vi "Create Arbitrary Waveform_Corr6.vi"(8 "error in (no error)":errorcluster, 10 "Waveform Name (\"wave1\")":string="wave1", 11 "VISA resource name":refnum<visa-resource-name>="USB0::0xF4EC::0x1101::SDG6XEBC5R0119::INSTR") -> ()   [LabVIEW 2018]
doc: "Creates and saves an arbitrary (user-defined) waveform in non-volatile memory, then selects it for output."
uses:
  <vilib>/Utility/file.llb/Read From Spreadsheet File (I64).vi
panel:
  out "error out":errorcluster
  out "VISA resource name out":refnum<visa-resource-name>
  out "Attempts":i32
  in  "WFM Source":u16(ring) items=["Single file", "Split files", "Array"]
  in  "WFM Path":path=path "C:/Data/_SoftDevelopment/SDG6000/PMHtst.txt"
  in  "WFM (Column) Number":i32
  in  "WFM Length":i32=15
  in  "Arbitrary Numeric Waveform Data":dbl[](array[numeric])=[1000.0, 2000.0, 3000.0, 4000.0, 5000.0, 6000.0, 7000.0, 8000.0]
  # "Same vi as with suppliers example,\nbut incorrect negativ case removed.\nInstead calculating twos complement\nexplicitly for negative values.\nThe input range for ARB data is\n-32768..+32767"
  # "C1 hardcoded as needs to have a channel assigned to be uploaded. \nCan then be used for either channel"
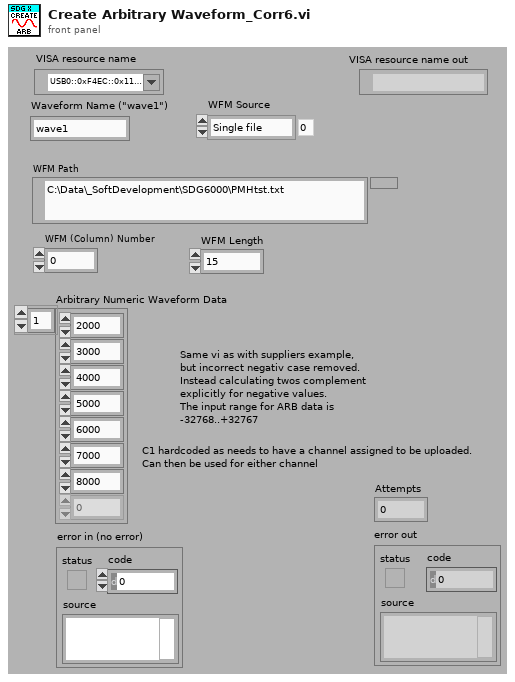
[diagram p1: front panel]
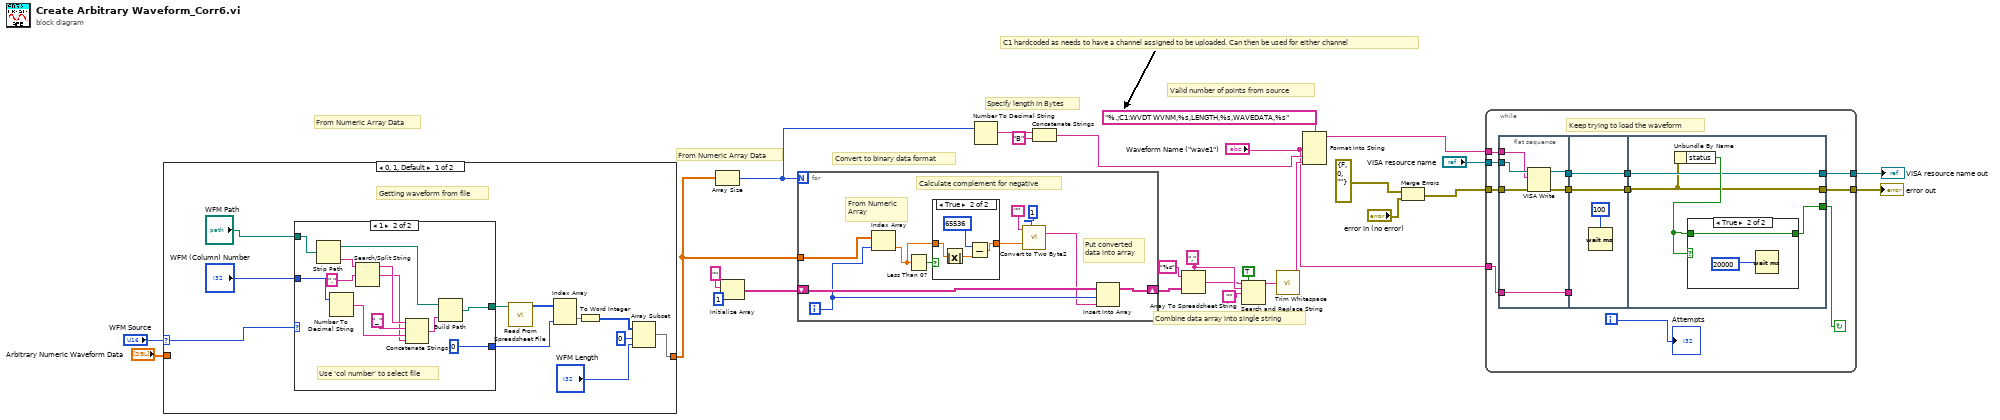
[diagram p0: block diagram]
diagram:
  w19 = ","
  # "C1 hardcoded as needs to have a channel assigned to be uploaded. Can then be used for either channel"
  # "From Numeric Array Data"
  # "From Numeric Array Data"
  # "Specify length in Bytes"
  # "Combine data array into single string"
  # "Valid number of points from source"
  # "Convert to binary data format"
  n1 = case shown="0, 1, Default" "WFM Source" {
    selector: "WFM Source" -> [w33 _]
    tunnel: [w28 w53] -> w8
    tunnel: "Arbitrary Numeric Waveform Data" -> [_ w53]
    frame 0, 1, Default {
      # "Getting waveform from file"
      n2 = case shown="1" w33 {
        tunnel: "WFM Path" -> [w40 w52]
        tunnel: "WFM (Column) Number" -> [w39 w49]
        tunnel: [w40 w42] -> w31
        tunnel: [w39 0 ("x")] -> w30
        frame 0, Default {
          # "File contains multiple wfms"
        }
        frame 1 {
          # "Use 'col number' to select file"
          n3 = Strip Path(path=w52) -> (stripped path=w44:path, name=w50:string)
          n4 = Number To Decimal String(number=w49) -> (decimal integer string=w46:string)  [unwired: 1 in]
          n5 = Search/Split String(string=w50, search string/char (-)=".") -> (substring before match=w48:string, match + rest of string=w45:string)  [unwired: 1 in, 1 out]
          n6 = Concatenate Strings(w48, "_", w46, w45) -> (w43:string)
          n7 = Build Path(base path=w44, name or relative path=w43) -> (appended path=w42:path)
        }
      }
      n8 = call-poly <vilib>:"Read From Spreadsheet File.vi"("file path (dialog if empty)"=w31) -> ("all rows"=w32:i64[][])  [unwired: 6 in, 4 out]
      n9 = Index Array(array=w32, index (col)=w30) -> (element=w29:i64[])  [unwired: 1 in]
      n10 = To Word Integer(number=w29) -> (16bit integer=w38:i16[])
      n11 = Array Subset(array=w38, index=0 ("x"), length="WFM Length") -> (w28:i16[])
    }
    frame 2 {
      # "Arbitrary Numeric Waveform Data"
    }
  }
  n12 = Array Size(array=w8) -> (size(s)=w26:i32)
  n13 = Initialize Array("", 1) -> (w23:string[])
  n14 = for {
    N: w26 -> [_]
    tunnel: w8 -> [w61]
    shift-right: [w57] -> w12
    shift-left: w23 -> [w60]
    i -> [w59]
    # "Calculate complement for negative"
    # "From Numeric\nArray"
    # "Put converted\ndata into array"
    n15 = Index Array(array=w61, index=w59) -> (element=w55:dbl)
    n16 = Less Than 0?(x=w55) -> (x < 0?=w56:bool)
    n17 = case shown="True" w56 {
      tunnel: w55 -> [w64 w65]
      tunnel: [w64 w68] -> w54
      frame False {
      }
      frame True {
        n18 = Absolute Value(x=w65) -> (abs(x)=w66:dbl)
        n19 = Subtract(x=65536, y=w66) -> (x-y=w68:dbl)
      }
    }
    n20 = call "Convert to Two Byte2.vi"("Input Method (0:String)"=u16 1, "Input Number"=w54, "Numeric String"="") -> ("Output String"=w58:string)  [unwired: 8 in]
    n21 = Insert Into Array(array=w60, index=w59, new element=w58) -> (w57:string[])
  }
  n22 = Number To Decimal String(number=w26) -> (decimal integer string=w15:string)  [unwired: 1 in]
  n23 = Concatenate Strings(w15, "B" ("string")) -> (w13:string)
  n24 = Array To Spreadsheet String(delimiter (Tab)=w19, array=w12, 3:"%s") -> (spreadsheet string=w16:string)
  n25 = Search and Replace String(replace all?=TRUE, input string=w16, search string=w19, replace string="") -> (result string=w17:string)  [unwired: 4 in, 3 out]
  n26 = call <vilib>:"Trim Whitespace.vi"("string"=w17) -> ("trimmed string"=w11:string)  [unwired: 1 in]
  n27 = Format Into String(format string="%.;C1:WVDT WVNM,%s,LENGTH,%s,WAVEDATA,%s", "Waveform Name (\"wave1\")", w13, w11) -> (resulting string=w2:string)  [unwired: 2 in, 1 out]
  n28 = Merge Errors(errorcluster {"status"=FALSE, "code"=0, "source"=""} ("error constant"), "error in (no error)") -> (w3:errorcluster)
  n29 = while {
    tunnel: w2 -> [w81]
    tunnel: "VISA resource name" -> [w80]
    tunnel: w3 -> [w79]
    tunnel: [w78] -> w6
    tunnel: [w77] -> w7
    tunnel: "Waveform Name (\"wave1\")" -> [w72]
    i -> [w73]
    stop <- w76 continue-if-true
    # "Keep trying to load the waveform"
    n30 = flat-sequence {
      tunnel: [w83] -> w75
      tunnel: [w84] -> w74
      tunnel: [w82] -> w71
      tunnel: w80 -> [w86]
      tunnel: w79 -> [w87]
      tunnel: w81 -> [w85]
      tunnel: w72 -> [w82]
      tunnel: w75 -> [w88]
      tunnel: w74 -> [w89]
      tunnel: w71 -> [_]
      tunnel: [w89] -> w70
      tunnel: [w88] -> w69
      tunnel: [w92] -> w77
      tunnel: [w91] -> w78
      tunnel: [w93] -> w76
      tunnel: w70 -> [w92]
      tunnel: w69 -> [w91]
      frame #0 {
        n31 = VISA Write(VISA resource name=w86, write buffer=w85, error in (no error)=w87) -> (VISA resource name out=w84:refnum<visa-resource-name>, error out=w83:errorcluster)  [unwired: 1 out]
      }
      frame #1 {
        n32 = Wait (ms)(milliseconds to wait=100 ("x")) -> ()  [unwired: 1 out]
      }
      frame #2 {
        n33 = Unbundle By Name(w91) -> ("status"=w94:bool)
        n34 = case shown="True" w94 {
          tunnel: w94 -> [w95 w96]
          tunnel: [w95 w96] -> w93
          frame False {
          }
          frame True {
            n35 = Wait (ms)(milliseconds to wait=20000 ("x")) -> ()  [unwired: 1 out]
          }
        }
      }
    }
    "Attempts" <- w73
  }
  "VISA resource name out" <- w7
  "error out" <- w6
